vi "Get Selection List.vi"(8 "error in (no error)":errorcluster, 11 "Search in":refnum<class "Search.lvclass">) -> (0 "error out":errorcluster, 2 "SelList[]":refnum<vi>[](array[refnum]), 3 "Search out":refnum<class "Search.lvclass">)   [LabVIEW 2016, in "Better Search.lvlib" / "Search.lvclass"]
uses:
  Search.lvclass
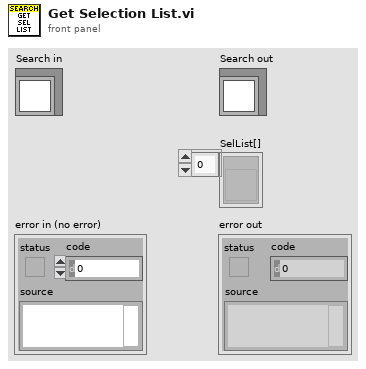
[diagram p1: front panel]
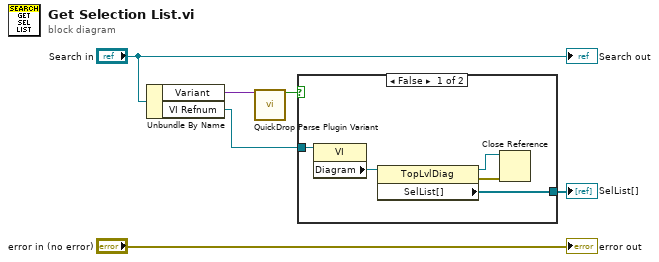
[diagram p0: block diagram]
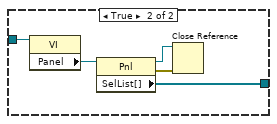
[diagram p2: hidden frame]
diagram:
  n1 = Unbundle By Name("Search in") -> ("Variant"=w4:variant, "VI Refnum"=w2:refnum<vi>)
  n2 = call <vilib>:"QuickDrop Parse Plugin Variant.vi"("QDKS Variant in"=w4) -> ("QD Launch VI Panel?"=w3:bool)  [unwired: 12 in, 2 out]
  n3 = case shown="False" w3 {
    tunnel: w2 -> [w11 w16]
    tunnel: [w9 w14] -> w1
    frame False {
      n4 = property class="VI"(reference=w11) -> ("Diagram"=w10:refnum<vi>)  [unwired: 1 in, 2 out]
      n5 = property class="TopLvlDiag"(reference=w10) -> (reference out=w7:refnum<vi>, error out=w8:errorcluster, "SelList[]"=w9:refnum<vi>[])  [unwired: 1 in]
      n6 = Close Reference(reference=w7, error in (no error)=w8) -> ()  [unwired: 1 out]
    }
    frame True {
      n7 = property class="VI"(reference=w16) -> ("Panel"=w15:refnum<vi>)  [unwired: 1 in, 2 out]
      n8 = property class="Pnl"(reference=w15) -> (reference out=w12:refnum<vi>, error out=w13:errorcluster, "SelList[]"=w14:refnum<vi>[])  [unwired: 1 in]
      n9 = Close Reference(reference=w12, error in (no error)=w13) -> ()  [unwired: 1 out]
    }
  }
  "SelList[]" <- w1
  "error out" <- "error in (no error)"
  "Search out" <- "Search in"
